vi "wavew.vi"() -> ()   [LabVIEW 2020]
uses:
  <vilib>/numeric/Random Number (Range) U64.vi
  <vilib>/numeric/sub_Random U32.vi
panel:
  in  "stop":bool
  out "Strip Chart":u64(graph)
  out "Sweep Chart 3":u64(graph)
  out "Scope Chart 2":u64(graph)
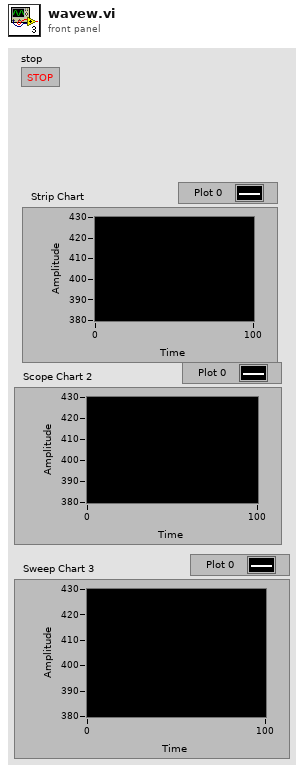
[diagram p1: front panel]
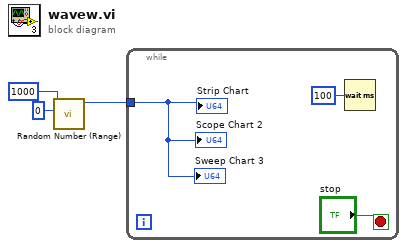
[diagram p0: block diagram]
diagram:
  n1 = call-poly <vilib>:"Random Number (Range).vi"("lower bound (0)"=u64 0, "upper bound (100)"=u64 1000) -> ("number"=w1:u64)  [unwired: 9 in]
  n2 = while {
    tunnel: w1 -> [w6]
    stop <- "stop" stop-if-true
    n3 = Wait (ms)(milliseconds to wait=u32 100) -> ()  [unwired: 1 out]
    "Scope Chart 2" <- w6
    "Sweep Chart 3" <- w6
    "Strip Chart" <- w6
  }
